vi "DFD Remez Order Estimation.vi"(6 "fs [Hz]":dbl=1.0 format="%.2f", 7 "filter type":T4(ring), 8 "error in (no error)":errorcluster, 9 "order option":enum16{"MinNum", "MinEven", "MinOdd"}(ring)=enum."MinEven", 10 "ripple specs":T1={"passband"=0.1, "stopband"=60.0, "dB/linear? (T: dB)"=TRUE}, 11 "freq specs [Hz]":T2={"fpass 1"=0.2, "fstop 1"=0.3, "fpass 2 "=0.0, "fstop 2"=0.0}) -> (0 "error out":errorcluster, 2 "band specs":T3[](array[typedef]), 3 "estimated order":i32)   [LabVIEW 2017, in "NI_DigFilterLicensed.lvlib"]
doc: "Estimates the order of a Remez equi-ripple filter."
uses:
  <vilib>/addons/Digital Filter Design/NI_DigFilterLicensed.lvlib
  <vilib>/addons/Digital Filter Design/_Objects.llb/DFD Adv Band Spec.ctl
  <vilib>/addons/Digital Filter Design/_Objects.llb/DFD Filter Frequence Specification (Design).ctl
  <vilib>/addons/Digital Filter Design/_Objects.llb/DFD Filter Ripple Specification (Design).ctl
panel:
  # "freq"
  # "amplitude"
  # "weight"
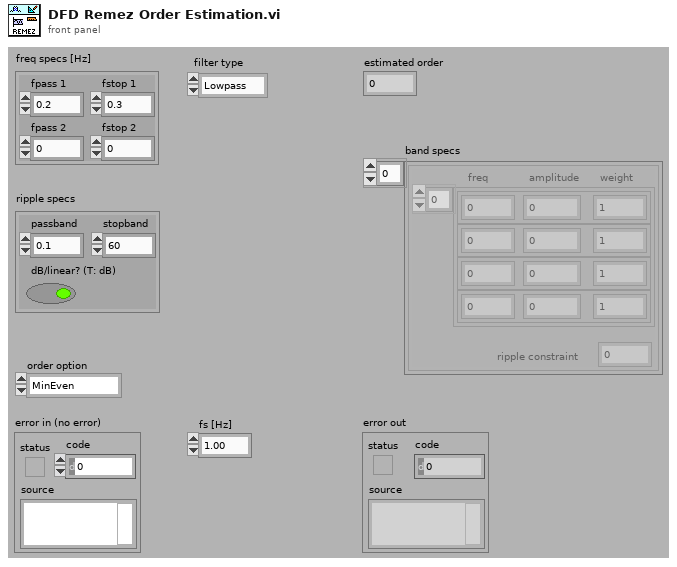
[diagram p1: front panel]
types:
  T1 = typedef "NI_DigFilterLicensed.lvlib/DFD Filter Ripple Specification (Design).ctl" = cluster{"passband":dbl, "stopband":dbl, "dB/linear? (T: dB)":bool}
  T2 = typedef "NI_DigFilterLicensed.lvlib/DFD Filter Frequence Specification (Design).ctl" = cluster{"fpass 1":dbl, "fstop 1":dbl, "fpass 2 ":dbl, "fstop 2":dbl}
  T3 = typedef "NI_DigFilterLicensed.lvlib/DFD Adv Band Spec.ctl" = cluster{"band specification":cluster{"freq":dbl, "amplitude":dbl, "weight":dbl}[], "ripple constraint":dbl}
  T4 = enum16{"Lowpass", "Highpass", "Bandpass", "Bandstop"}
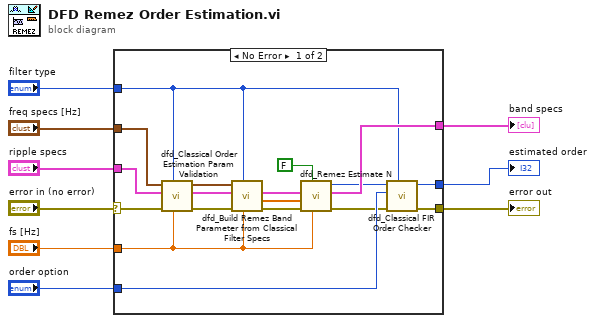
[diagram p0: block diagram]
diagram:
  n1 = case shown="No Error" "error in (no error)" {
    selector: "error in (no error)" -> [w10 w28]
    tunnel: [w27 w28] -> w9
    tunnel: [w26 _] -> w8
    tunnel: "order option" -> [w25 _]
    tunnel: "fs [Hz]" -> [w23 _]
    tunnel: [w22 _] -> w5
    tunnel: "filter type" -> [w21 _]
    tunnel: "freq specs [Hz]" -> [w14 _]
    tunnel: "ripple specs" -> [w12 _]
    frame No Error {
      n2 = call <vilib>:"dfd_Classical Order Estimation Param Validation.vi"("fs [Hz]"=w23, "filter type"=w21, "error in (no error)"=w10, "ripple specs"=w12, "freq specs [Hz]"=w14) -> ("error out"=w24:errorcluster, "dup ripple specs"=w11:T1, "dup freq specs [Hz]"=w13:T2)  [unwired: 1 in, 3 out]
      n3 = call <vilib>:"dfd_Build Remez Band Parameter from Classical Filter Specs.vi"("fs [Hz]"=w23, "filter type"=w21, "error in (no error)"=w24, "ripple specs"=w11, "freq specs [Hz]"=w13) -> ("error out"=w19:errorcluster, "band ripples"=w20:dbl[], "band parameters"=w16:T3[])  [unwired: 4 out]
      n4 = call <vilib>:"dfd_Remez Estimate N.vi"("fs [Hz]"=w23, "auto order"=FALSE ("set constrain"), "error in (no error)"=w19, "band ripple"=w20, "band parameters"=w16) -> ("error out"=w18:errorcluster, "band parameters dup"=w22:T3[], "estimated order"=w17:i32)  [unwired: 4 out]
      n5 = call <vilib>:"dfd_Classical FIR Order Checker.vi"("filter type"=w21, "error in (no error)"=w18, "order option"=w25, "order in"=w17) -> ("error out"=w27:errorcluster, "order out"=w26:i32)  [unwired: 6 out]
    }
    frame Error {
    }
  }
  "error out" <- w9
  "estimated order" <- w8
  "band specs" <- w5
